vi "rohitCALC.vi"() -> ()   [LabVIEW 2009]
panel:
  in  "Enum":T1(ring)
  out "Numeric 3":dbl
  in  "Numeric 2":dbl
  in  "Numeric":dbl
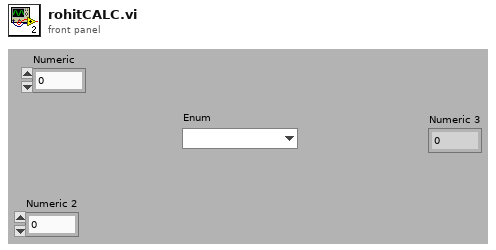
[diagram p1: front panel]
types:
  T1 = enum16{"", "ADD", "SUBTRACT", "DIVIDE", "MULTIPLY"}
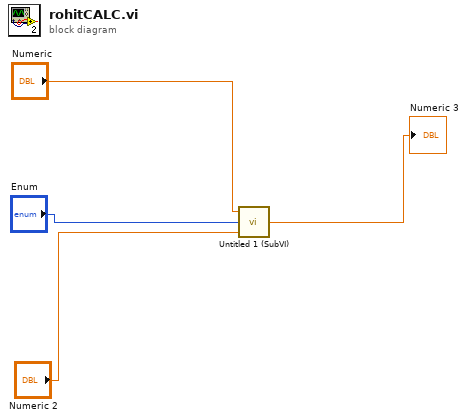
[diagram p0: block diagram]
diagram:
  n1 = call "Untitled 1 (SubVI).vi"("Numeric 2"="Numeric 2", "Enum"="Enum", "Numeric"="Numeric") -> ("Numeric 3"=→"Numeric 3":dbl)
